vi "SHift to time.vi"() -> ()   [LabVIEW 2017]
panel:
  out "time stamp":timestamp
  in  "Date":timestamp format="%<%Y-%m-%d>T"
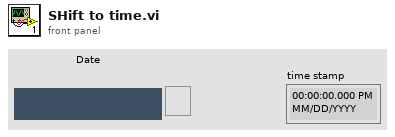
[diagram p1: front panel]
types:
  T1 = typedef "LVDateTimeRec.ctl" = cluster{"fractional second":dbl, "second":i32, "minute":i32, "hour":i32, "day of month":i32, "month":i32, "year":i32, "day of week":i32, "day of year":i32, "DST":i32}
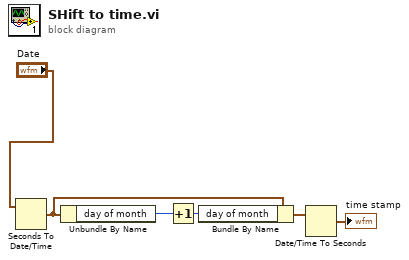
[diagram p0: block diagram]
diagram:
  n1 = Seconds To Date/Time(time stamp (now)="Date") -> (date time rec=w2:T1)  [unwired: 1 in]
  n2 = Unbundle By Name(w2) -> ("day of month"=w4:i32)
  n3 = Increment(x=w4) -> (x+1=w5:i32)
  n4 = Bundle By Name(cluster=w2, "day of month"=w5) -> (w6:T1)
  n5 = Date/Time To Seconds(2:w6) -> (0:→"time stamp":timestamp)  [unwired: 1 in]
